vi "Convert Clustered Arrays to Channels.vi"(8 "error in (no error)":errorcluster, 10 "[VData out]":variant[](array[variant]), 11 "[Parsed Tags]":T1[](array[typedef])) -> (0 "error out":errorcluster, 1 "[Whole Tags]":string[](array[string]), 2 "[VData out]":variant[](array[variant]), 3 "[Parsed Tags]":T1[](array[typedef]))   [LabVIEW 2018]
uses:
  Shared Controls/Parsed Tag Cluster.ctl
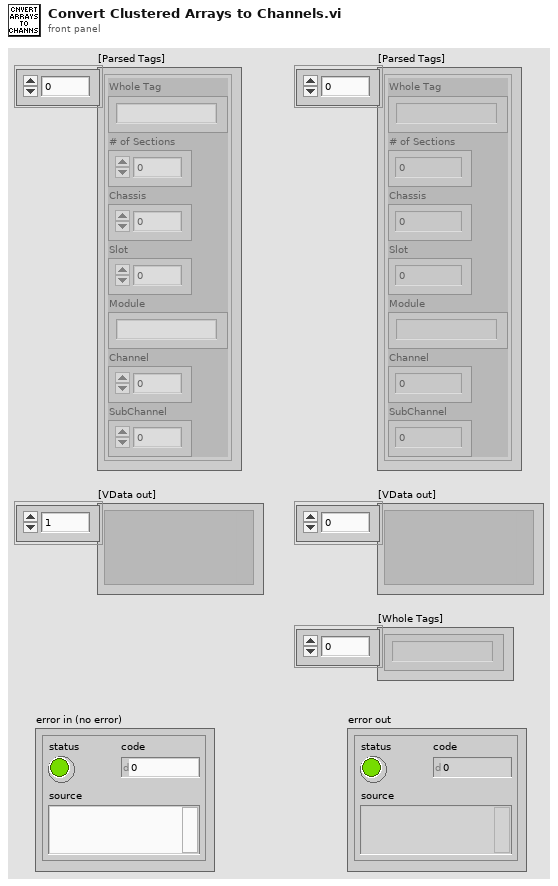
[diagram p1: front panel]
types:
  T1 = typedef "Parsed Tag Cluster.ctl" = cluster{"Whole Tag":string, "# of Sections":u8, "Chassis":u8, "Slot":u8, "Module":string, "Channel":u8, "SubChannel":u8}
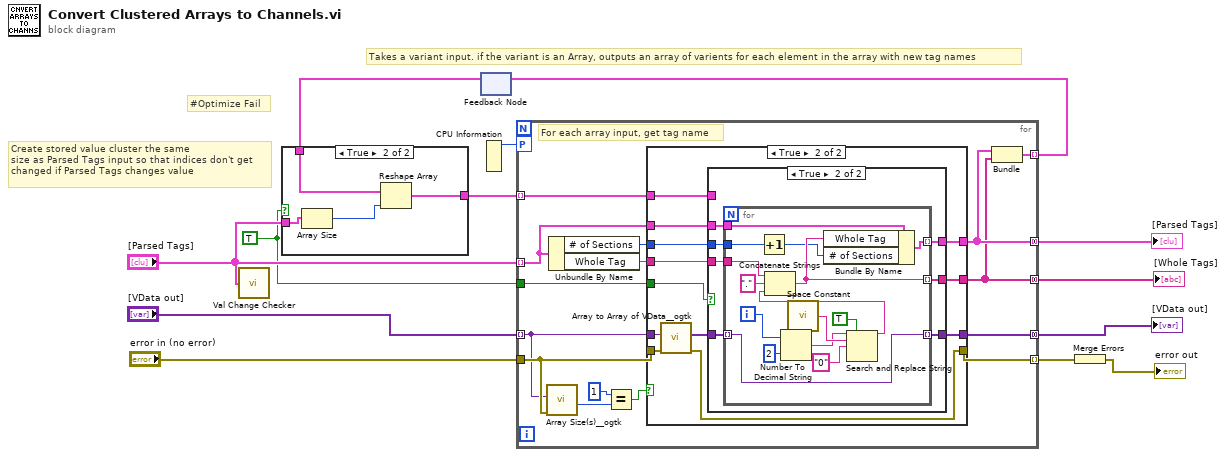
[diagram p0: block diagram]
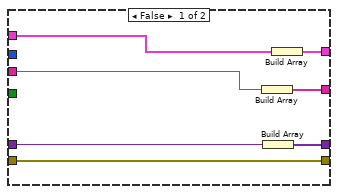
[diagram p3: hidden frame]
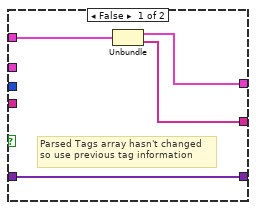
[diagram p4: hidden frame]
diagram:
  w1 = TRUE ("Value Change?")
  # "#Optimize Fail"
  # "Create stored value cluster the same\nsize as Parsed Tags input so that indices don't get\nchanged if Parsed Tags changes value"
  # "Takes a variant input. if the variant is an Array, outputs an array of varients for each element in the array with new tag names"
  n1 = call "Val Change Checker.vi"("Current Value in"="[Parsed Tags]") -> ()  [unwired: 1 out]
  n2 = CPU Information() -> (4:w6:i32)  [unwired: 3 out]
  n3 = feedback #1() -> (w4:cluster{T1[], string[]}[])  [unwired: 1 in]
  n4 = case shown="True" w1 {
    tunnel: "[Parsed Tags]" -> [_ w18]
    tunnel: w4 -> [w14 w17]
    tunnel: [w14 w15] -> w2
    frame False {
    }
    frame True {
      n5 = Array Size(array=w18) -> (size(s)=w16:i32)
      n6 = Reshape Array(w17, w16) -> (w15:cluster{T1[], string[]}[])
    }
  }
  n7 = for {
    tunnel: "[Parsed Tags]" -> [w32] mode=indexing
    tunnel: "[VData out]" -> [w25] mode=indexing
    tunnel: "error in (no error)" -> [w26]
    tunnel: [w33] -> w8 mode=indexing
    tunnel: [w22] -> w11 mode=concatenating
    tunnel: [w30] -> w12 mode=concatenating
    tunnel: [w21] -> w13 mode=concatenating
    workers-P: w6 -> [_]
    tunnel: w1 -> [w23]
    tunnel: [w20] -> w3 mode=indexing
    tunnel: w2 -> [w19] mode=indexing
    # "For each array input, get tag name"
    n8 = call <userlib>:"Array Size(s)__ogtk.vi"("error in (no error)"=w26, "Array"=w25) -> ("N dims"=w28:u32)  [unwired: 7 in, 2 out]
    n9 = Unbundle By Name(w32) -> ("# of Sections"=w24:u8, "Whole Tag"=w31:string)
    n10 = Equal?(x=u32 1, y=w28) -> (x = y?=w29:bool)
    n11 = case shown="True" w29 {
      tunnel: w26 -> [w35 w52]
      tunnel: [w35 w48] -> w33
      tunnel: w25 -> [w39 w51]
      tunnel: w32 -> [w34 w49]
      tunnel: [w40 w47] -> w22
      tunnel: [w37 w46] -> w21
      tunnel: w31 -> [w38 w50]
      tunnel: [w36 w45] -> w30
      tunnel: w24 -> [_ w44]
      tunnel: w23 -> [_ w42]
      tunnel: w19 -> [_ w41]
      frame False {
        n12 = Build Array(w38) -> (w37:string[])
        n13 = Build Array(w39) -> (w36:variant[])
        n14 = Build Array(w34) -> (w40:T1[])
      }
      frame True {
        n15 = call <userlib>:"Array to Array of VData__ogtk.vi"("error in (no error)"=w52, "MultiD Array"=w51) -> ("error out"=w48:errorcluster, "1D Array of Variants"=w43:variant[])  [unwired: 8 in]
        n16 = case shown="True" w42 {
          tunnel: w50 -> [_ w63]
          tunnel: w49 -> [_ w62]
          tunnel: [w54 w61] -> w47
          tunnel: [w53 w60] -> w46
          tunnel: [w56 w59] -> w45
          tunnel: w44 -> [_ w58]
          tunnel: w43 -> [w56 w57]
          tunnel: w41 -> [w55 _]
          frame False {
            # "Parsed Tags array hasn't changed\nso use previous tag information"
            n17 = Unbundle(w55) -> (w54:T1[], w53:string[])
          }
          frame True {
            n18 = for {
              tunnel: w63 -> [w70]
              tunnel: w62 -> [w69]
              tunnel: w57 -> [w66] mode=indexing
              tunnel: [w68] -> w61 mode=indexing
              tunnel: [w67] -> w60 mode=indexing
              tunnel: [w66] -> w59 mode=indexing
              tunnel: w58 -> [w65]
              i -> [w73]
              n19 = Increment(x=w65) -> (x+1=w64:u8)
              n20 = Number To Decimal String(number=w73, width (-)=i16 2) -> (decimal integer string=w75:string)
              n21 = call <vilib>:"Space Constant.vi"() -> ("String"=w76:string)
              n22 = Search and Replace String(replace all?=TRUE ("replace all? (F)"), input string=w75, search string=w76, replace string="0" ("replace string (\"\")")) -> (result string=w71:string)  [unwired: 4 in, 3 out]
              n23 = Concatenate Strings(w70, "." ("string"), w71) -> (w67:string)
              n24 = Bundle By Name(cluster=w69, "Whole Tag"=w67, "# of Sections"=w64) -> (w68:T1)
            }
          }
        }
      }
    }
    n25 = Bundle(w22, w21) -> (w20:cluster{T1[], string[]})  [unwired: 1 in]
  }
  "[Whole Tags]" <- w13
  "[VData out]" <- w12
  "[Parsed Tags]" <- w11
  n26 = feedback-in #1(w3) -> ()
  n27 = Merge Errors(w8) -> (→"error out":errorcluster)
